vi "PH_SHS_Analysis_Calibrator.set GUI elements.vi"(0 "i ref in":refnum<vi>, 1 "ok visible (true)":bool=TRUE, 2 "skip visible (true)":bool=TRUE, 3 "Repeat visible (true)":bool=TRUE, 4 "Cancel visible (true)":bool=TRUE, 5 "error in (no error)":errorcluster, 6 "Cams disabled (true)":bool=TRUE) -> (14 "i ref out":refnum<vi>, 19 "error out":errorcluster)   [LabVIEW 2014, in "PH_SHS_Analysis_Calibrator.lvlib"]
doc: "This VI sets the GUI elements to be visible (resp. grayed out)"
uses:
  PH_SHS_Analysis_Calibrator.lvlib
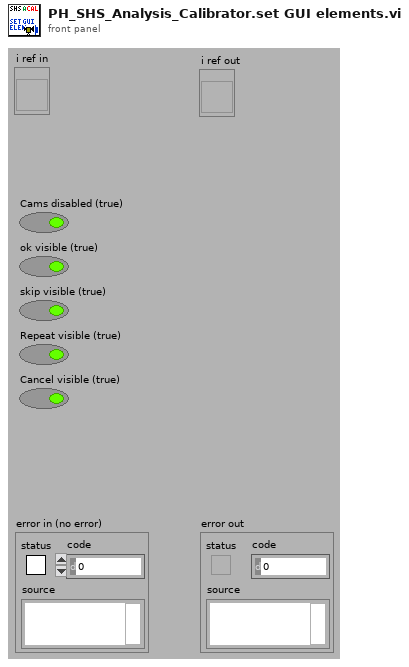
[diagram p1: front panel]
types:
  T1 = typedef "PH_SHS_Analysis_Calibrator.lvlib/PH_SHS_Analysis_Calibrator.i attribute.ctl" = cluster{"GUI Refs":cluster{"Available Cams":refnum<vi>, "OK":refnum<vi>, "Skip":refnum<vi>, "Repeat":refnum<vi>, "Cancel":refnum<vi>, "Dialog":refnum<vi>, "Enough Images?":refnum<vi>}, "Cam instances":string[], "Status":cluster{"#":i32, "Data calculated":bool, "Wanted #":i32}, "IMAQ Image Array":T2[], "Pixel Size [µm]":dbl, "MLA Pitch [µm]":dbl, "Method":enum16{"automatic", "manual"}, "Enough Images?":bool, "SHS Reference Result":T3, "Calculation Error":errorcluster}
  T2 = typedef "IMAQ Image.ctl" = refnum<image>
  T3 = typedef "SHS_Common.lvlib/SHSReference.ctl" = cluster{"Reference":T4[][], "Lens Array Pitch [px]":dbl}
  T4 = typedef "SHS_Common.lvlib/ReferencePoint.ctl" = cluster{"Rect":T5, "Point":T6}
  T5 = typedef "SHS_Common.lvlib/Rectangle.ctl" = cluster{"Left":i32, "Top":i32, "Right":i32, "Bottom":i32}
  T6 = typedef "SHS_Common.lvlib/Point.ctl" = cluster{"x":dbl, "y":dbl, "valid?":bool, "weight":dbl}
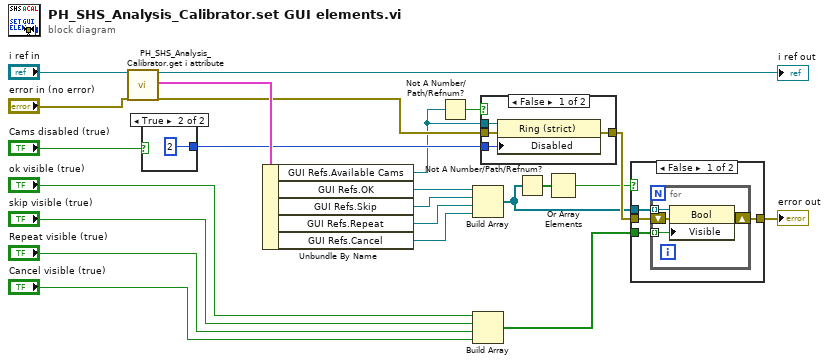
[diagram p0: block diagram]
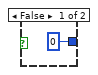
[diagram p4: hidden frame]
diagram:
  n1 = call "PH_SHS_Analysis_Calibrator.get i attribute.vi"("i ref in"="i ref in", "error in (no error)"="error in (no error)") -> ("i ref out"=→"i ref out":refnum<vi>, "i attribute"=w20:T1, "error out"=w12:errorcluster)  [unwired: 15 in]
  n2 = case shown="True" "Cams disabled (true)" {
    tunnel: [u8 0 ("Disabled") u8 2 ("Disabled")] -> w19
    frame False {
    }
    frame True {
    }
  }
  n3 = Unbundle By Name(w20) -> ("GUI Refs.Available Cams"=w10:refnum<vi>, "GUI Refs.OK"=w14:refnum<vi>, "GUI Refs.Skip"=w15:refnum<vi>, "GUI Refs.Repeat"=w16:refnum<vi>, "GUI Refs.Cancel"=w17:refnum<vi>)
  n4 = Not A Number/Path/Refnum?(number/path/refnum=w10) -> (NaN/Path/Refnum?=w11:bool)
  n5 = Build Array(w14, w15, w16, w17) -> (w7:refnum<vi>[])
  n6 = Build Array("ok visible (true)", "skip visible (true)", "Repeat visible (true)", "Cancel visible (true)") -> (w8:bool[])
  n7 = case shown="False" w11 {
    tunnel: w10 -> [w29 _]
    tunnel: w19 -> [w28 _]
    tunnel: w12 -> [w27 w30]
    tunnel: [w26 w30] -> w9
    frame False {
      n8 = property class="Ring (strict)"(reference=w29, error in=w27, "Disabled"=w28) -> (error out=w26:errorcluster)  [unwired: 1 out]
    }
    frame True {
    }
  }
  n9 = Not A Number/Path/Refnum?(number/path/refnum=w7) -> (NaN/Path/Refnum?=w6:bool[])
  n10 = Or Array Elements(Boolean array=w6) -> (logical OR=w5:bool)
  n11 = case shown="False" w5 {
    tunnel: [w34 w39] -> w1
    tunnel: w9 -> [w33 w39]
    tunnel: w7 -> [w32 _]
    tunnel: w8 -> [w31 _]
    frame False {
      n12 = for {
        shift-right: [w38] -> w34
        shift-left: w33 -> [w37]
        tunnel: w32 -> [w36] mode=indexing
        tunnel: w31 -> [w35] mode=indexing
        n13 = property class="Bool"(reference=w36, error in=w37, "Visible"=w35) -> (error out=w38:errorcluster)  [unwired: 1 out]
      }
    }
    frame True {
    }
  }
  "error out" <- w1
